vi "Command Toggle Can Grabber.vi"(2 "Input Robot System Funtions":T1, 3 "Cmd Parameter 1":dbl, 4 "Cmd Parameter 2":dbl, 5 "Startup":bool) -> (0 "Output Robot System Functions":T1, 1 "Completed":bool)   [LabVIEW 2014]
uses:
  Subsystems VIs/Robot Commands.ctl
  Command Execution State.ctl
panel:
  # "Sample robot\ncontrol output.\nReplace with \nactual teleop \ncontrol signal \nstructure."
  # "Field Centric"
  # "Field Centric"
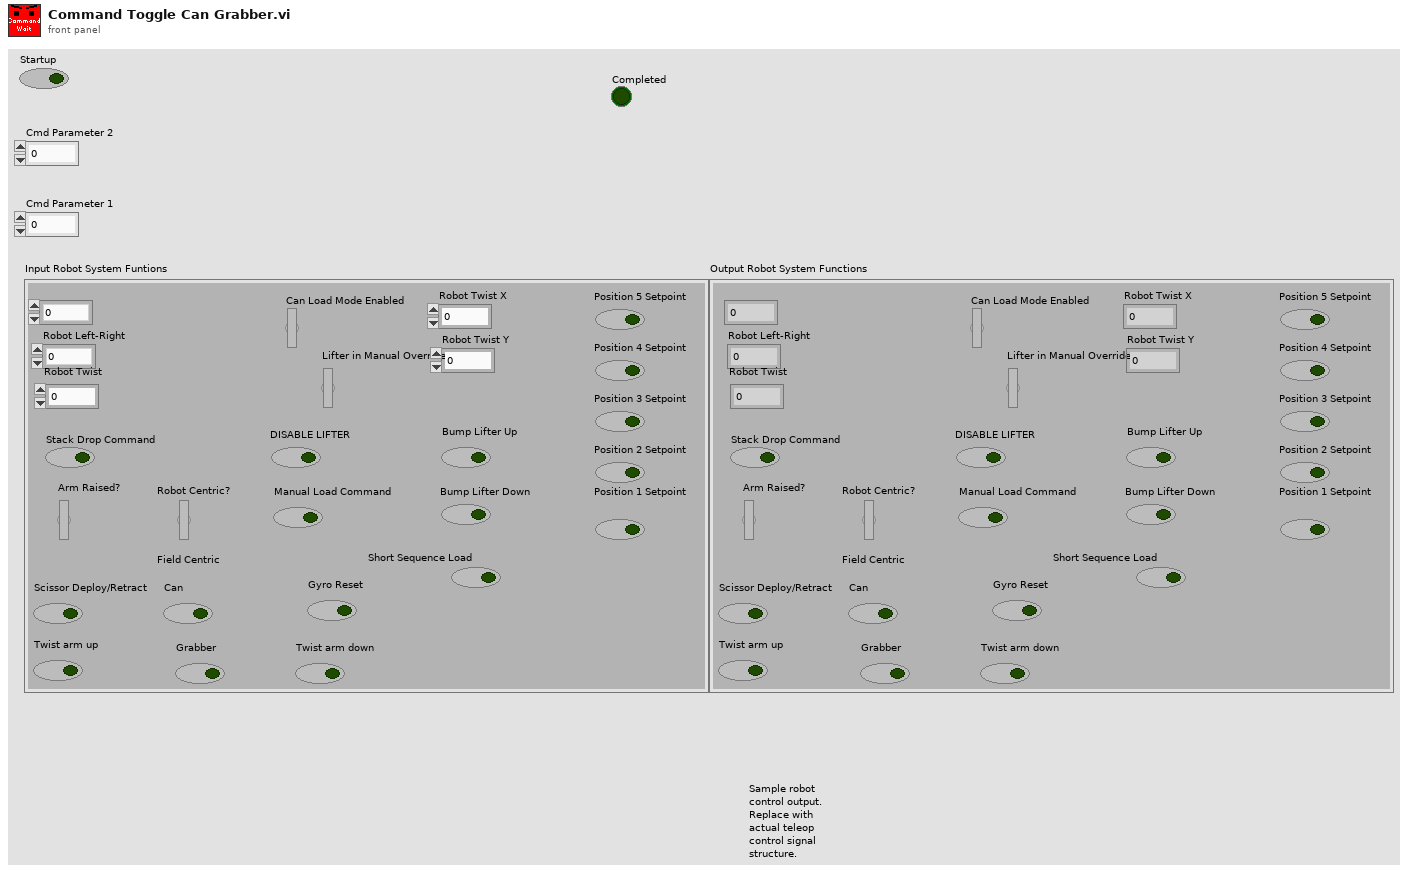
[diagram p1: front panel]
types:
  T1 = typedef "Robot Commands.ctl" = cluster{"Robot Forward-Reverse":dbl, "Robot Left-Right":dbl, "Robot Twist":dbl, "Can Load Mode Enabled":bool, "Lifter in Manual Override?":bool, "Stack Drop Command":bool, "Arm Raised?":bool, "DISABLE LIFTER":bool, "Position 1 Setpoint":bool, "Position 2 Setpoint":bool, "Position 3 Setpoint":bool, "Position 4 Setpoint":bool, "Position 5 Setpoint":bool, "Bump Lifter Down":bool, "Bump Lifter Up":bool, "Manual Load Command":bool, "Robot Centric?":bool, "Scissor Deploy/Retract":bool, "Grabber":bool, "Can":bool, "Twist arm up":bool, "Gyro Reset":bool, "Twist arm down":bool, "Short Sequence Load":bool, "Robot Twist X":dbl, "Robot Twist Y":dbl}
  T2 = typedef "Command Execution State.ctl" = enum16{"Initialize", "Execute", "Finish"}
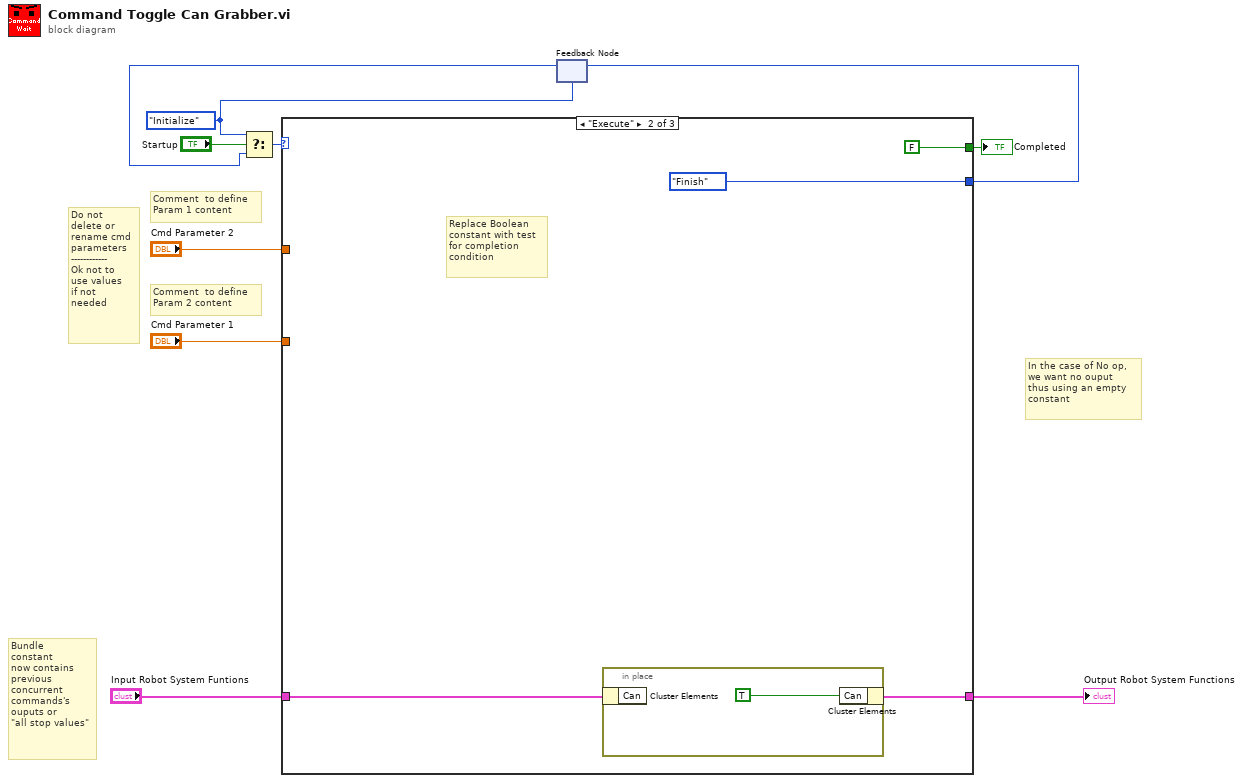
[diagram p0: block diagram]
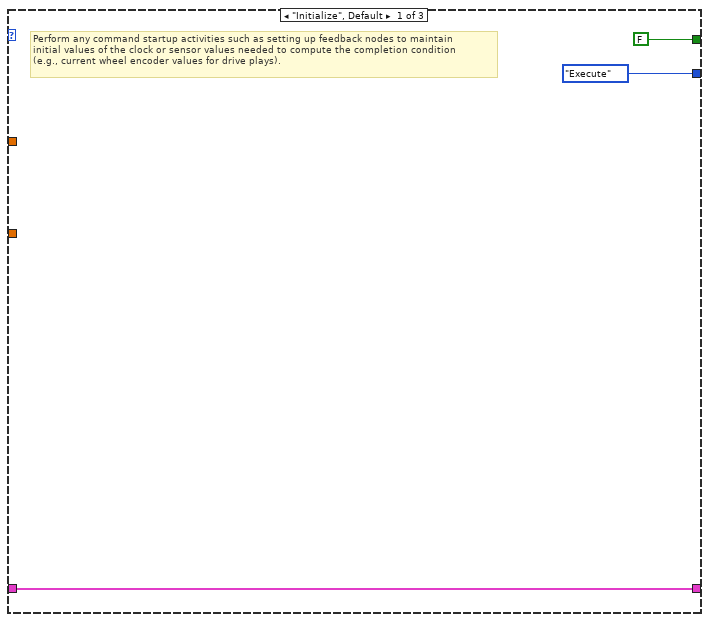
[diagram p2: hidden frame]
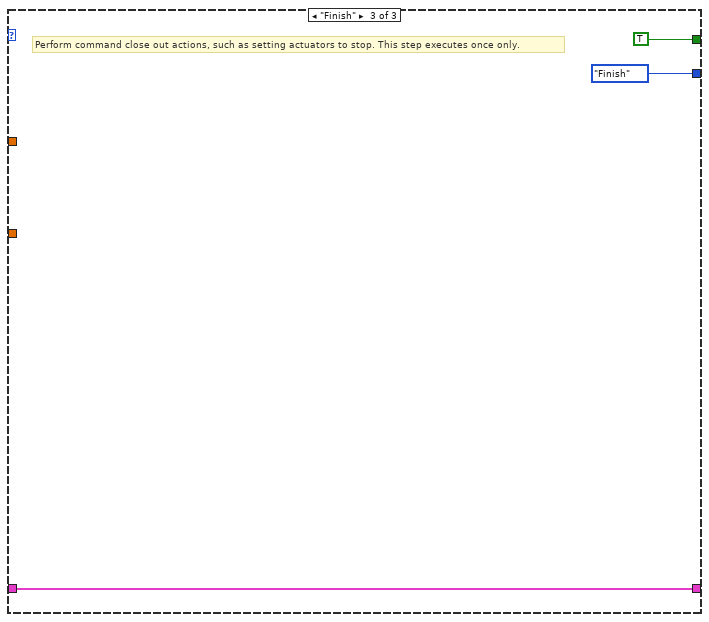
[diagram p3: hidden frame]
diagram:
  w5 = Command_Execution_State."Initialize" ("Play State")
  # "In the case of No op, \nwe want no ouput \nthus using an empty \nconstant"
  # "Bundle \nconstant\nnow contains\nprevious \nconcurrent\ncommands's\nouputs or\n\"all stop values\""
  # "Do not \ndelete or\nrename cmd\nparameters\n------------\nOk not to \nuse values\nif not \nneeded"
  # "Comment  to define\nParam 2 content"
  # "Comment  to define\nParam 1 content"
  n1 = feedback #1(w5) -> (w6:T2)
  n2 = Select(t=w5, s="Startup", f=w6) -> (s? t:f=w10:T2)
  n3 = case shown="\"Execute\"" w10 {
    tunnel: [FALSE FALSE TRUE] -> w8
    tunnel: [Command_Execution_State."Execute" ("Play State") Command_Execution_State."Finish" ("Play State") Command_Execution_State."Finish" ("f")] -> w7
    tunnel: "Cmd Parameter 2" -> [_ _ _]
    tunnel: "Cmd Parameter 1" -> [_ _ _]
    tunnel: [w11 w15 w19] -> w1
    tunnel: "Input Robot System Funtions" -> [w11 w16 w19]
    frame "Initialize", Default {
      # "Perform any command startup activities such as setting up feedback nodes to maintain \ninitial values of the clock or sensor values needed to compute the completion condition\n(e.g., current wheel encoder values for drive plays)."
    }
    frame "Execute" {
      # "Replace Boolean\nconstant with test \nfor completion \ncondition"
      n4 = in-place {
        n5 = in-place-cluster #2(w16) -> ()  [unwired: 1 out]
        n6 = in-place-cluster #2("Can"=TRUE ("Position 1 Setpoint")) -> (w15:T1)
      }
    }
    frame "Finish" {
      # "Perform command close out actions, such as setting actuators to stop. This step executes once only."
    }
  }
  "Completed" <- w8
  "Output Robot System Functions" <- w1
  n7 = feedback-in #1(w7) -> ()
